vi "Autonomous.vi"() -> ()   [LabVIEW 2017]
doc: "This VI starts when autonomous period begins, and will automatically be terminated when it ends. You can carry out timed or sensor driven operations directly to I/O or to subsystems without needing to return to the caller."
uses:
  Shared/AutoRoutineSelector.ctl
  ccd5ff82-f8db-4a3c-9200-aaa5681706e7.vi
  <vilib>/Rock Robotics/Network Tables/NT Read Number.vi
  <vilib>/Rock Robotics/Network Tables/NT Read Boolean.vi
  <vilib>/Rock Robotics/Network Tables/NT Read Numeric Array.vi
  <vilib>/Rock Robotics/Network Tables/NT Write String.vi
panel:
  out "File Path 4":string="3B.txt"
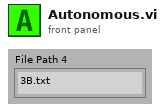
[diagram p1: front panel]
types:
  T1 = typedef "AutoRoutineSelector.ctl" = enum16{"Definately Switch", "Definately Scale", "Switch if in front, else scale", "Scale if in front, else switch", "Switch if in front, else cross line", "Scale if in front, else cross line", "Drive across line"}
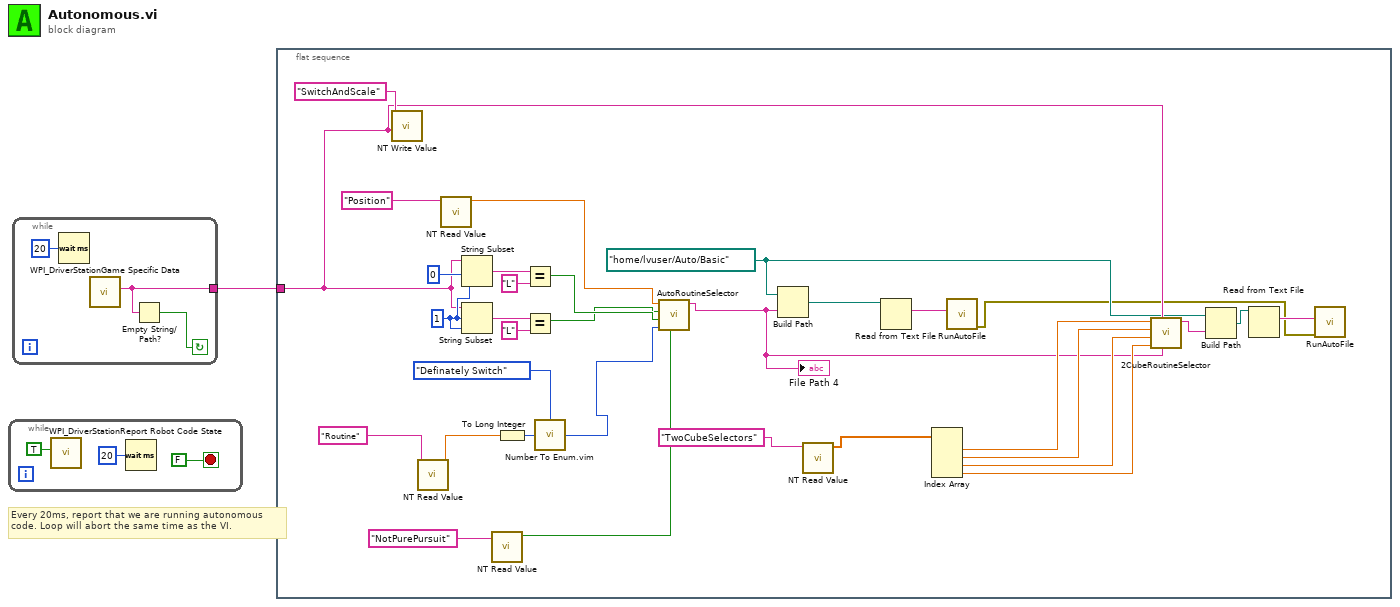
[diagram p0: block diagram]
diagram:
  # "Every 20ms, report that we are running autonomous\ncode. Loop will abort the same time as the VI."
  n1 = while {
    stop <- FALSE stop-if-true
    n2 = call <vilib>:"WPI_DriverStationReport Robot Code State.vi"("Autonomous"=TRUE) -> ()  [unwired: 10 in, 1 out]
    n3 = Wait (ms)(milliseconds to wait=u32 20) -> ()  [unwired: 1 out]
  }
  n4 = while {
    tunnel: [w7] -> w1
    stop <- w6 continue-if-true
    n5 = Wait (ms)(milliseconds to wait=u32 20) -> ()  [unwired: 1 out]
    n6 = call <vilib>:"WPI_DriverStationGame Specific Data.vi"() -> ("Game Specific Data"=w7:string)  [unwired: 11 in]
    n7 = Empty String/Path?(string/path=w7) -> (empty?=w6:bool)
  }
  n8 = flat-sequence {
    tunnel: w1 -> [w17]
    frame #0 {
      w14 = path "/home/lvuser/Auto/Basic" ("base path")
      w33 = 1 ("length (rest)")
      n9 = call-poly <vilib>:"NT Write Value.vi"("String"=w17, "Name"="SwitchAndScale") -> ()  [unwired: 9 in, 1 out]
      n10 = call-poly <vilib>:"NT Read Value.vi"("Name"="Routine") -> ("Numeric"=w39:dbl)  [unwired: 9 in, 1 out]
      n11 = call-poly <vilib>:"NT Read Value.vi"("Name"="Position") -> ("Numeric"=w8:dbl)  [unwired: 9 in, 1 out]
      n12 = String Subset(string=w17, offset (0)=0 ("length (rest)"), length (rest)=w33) -> (substring=w38:string)
      n13 = String Subset(string=w17, offset (0)=w33, length (rest)=w33) -> (substring=w37:string)
      n14 = call-poly <vilib>:"NT Read Value.vi"("Name"="NotPurePursuit") -> ("Boolean"=w9:bool)  [unwired: 9 in, 1 out]
      n15 = To Long Integer(number=w39) -> (32bit integer=w36:i32)
      n16 = Equal?(x=w38, y="L") -> (x = y?=w28:bool)
      n17 = Equal?(x=w37, y="L") -> (x = y?=w27:bool)
      n18 = call "Number To Enum.vim"("number"=w36, "enum type"=AutoRoutineSelector."Definately Switch" ("Routine")) -> ("number as enum"=w10:T1)
      n19 = call "AutoRoutineSelector.vi"("NotPurePursuit"=w9, "Routine"=w10, "OurSwitch"=w28, "OurScale"=w27, "Position"=w8) -> ("File Name"=w18:string)  [unwired: 6 in]
      "File Path 4" <- w18
      n20 = Build Path(base path=w14, name or relative path=w18) -> (appended path=w26:path)
      n21 = call-poly <vilib>:"NT Read Value.vi"("Name"="TwoCubeSelectors") -> ("Numeric Array"=w11:dbl[])  [unwired: 9 in, 1 out]
      n22 = Read from Text File(file (use dialog)=w26) -> (text=w25:string)  [unwired: 3 in, 3 out]
      n23 = Index Array(array=w11) -> (element #1=w22:dbl, element #2=w21:dbl, element #3=w20:dbl, element #4=w19:dbl)  [unwired: 4 in]
      n24 = call "RunAutoFile.vi"("AutoFile"=w25) -> ("error out"=w12:errorcluster)  [unwired: 10 in]
      n25 = call "2CubeRoutineSelector.vi"("Prior Routine File Name"=w18, "GameData"=w17, "ScaleOtherNotClose"=w19, "ScaleOtherClose"=w20, "SwitchOtherNotClose"=w21, "SwitchOtherClose"=w22) -> ("File Path"=w13:string)  [unwired: 5 in]
      n26 = Build Path(base path=w14, name or relative path=w13) -> (appended path=w15:path)
      n27 = Read from Text File(file (use dialog)=w15) -> (text=w16:string)  [unwired: 3 in, 3 out]
      n28 = call "RunAutoFile.vi"("error in (no error)"=w12, "AutoFile"=w16) -> ()  [unwired: 9 in, 1 out]
    }
  }
